vi "Pack For Grpc.vi"(7 "Results? (Config)":bool, 8 "error in (no error)":errorcluster, 10 "Data Value":variant, 11 "gRPCid":T2) -> (0 "error out":errorcluster, 2 "Any":T1)   [LabVIEW 2020, in "MeasurementLink Measurement Template.lvlib"]
uses:
  MeasurementLink Measurement Template.lvlib
  <vilib>/gRPC/LabVIEW gRPC Library/Shared/grpcId.ctl
  <vilib>/gRPC/LabVIEW gRPC Library/Shared/Any.ctl
  Measurement Results.ctl
  Measurement Configuration.ctl
  a6012965-5700-4384-8228-972e71b6560c.vi
  2eca732d-dbaa-43bf-a7dd-ede2da65bc1b.vi
  <vilib>/gRPC/LabVIEW gRPC Library/Server API/Translate Protobuf Error.vi
  <vilib>/AdvancedString/1D String Array to Delimited String.vi
  <vilib>/gRPC/LabVIEW gRPC Library/Server API/Server/Get Server DLL Path.vi
  <vilib>/gRPC/LabVIEW gRPC Library/grpc-lvsupport-release.lvlib
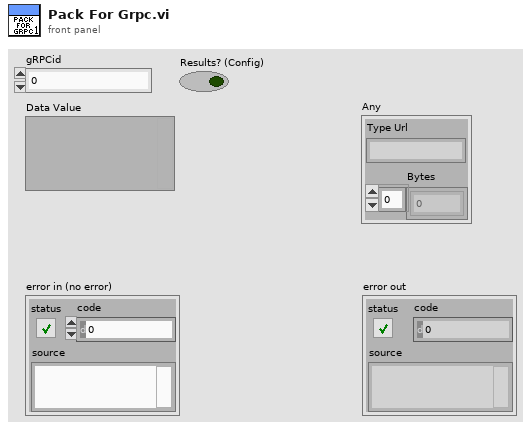
[diagram p1: front panel]
types:
  T1 = typedef "grpc-lvsupport-release.lvlib/Any.ctl" = cluster{"Type Url":string, "Bytes":u8[]}
  T2 = typedef "grpc-lvsupport-release.lvlib/grpcId.ctl" = u64
  T3 = typedef "MeasurementLink Measurement Template.lvlib/Measurement Results.ctl" = cluster{"Array out":dbl[]}
  T4 = typedef "MeasurementLink Measurement Template.lvlib/Measurement Configuration.ctl" = cluster{"Array in":dbl[]}
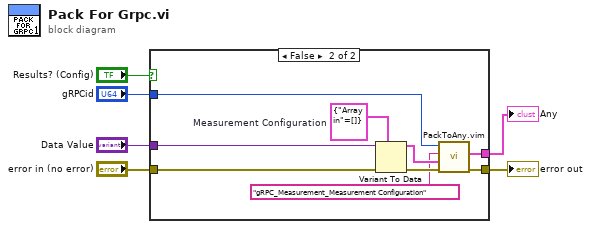
[diagram p0: block diagram]
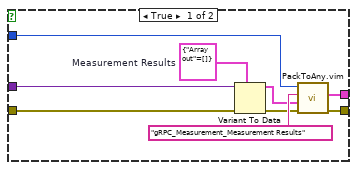
[diagram p2: hidden frame]
diagram:
  n1 = case shown="False" "Results? (Config)" {
    tunnel: "error in (no error)" -> [w15 w24]
    tunnel: "Data Value" -> [w14 w23]
    tunnel: "gRPCid" -> [w10 w20]
    tunnel: [w12 w22] -> w3
    tunnel: [w11 w21] -> w2
    frame True {
      w13 = T3 {"Array out"=[]}  # Measurement Results
      n2 = Variant To Data(error in=w15, type=w13, Variant=w14) -> (data=w8:T3, error out=w7:errorcluster)
      n3 = call "PackToAny.vim"("error in"=w7, "Data To Pack"=w8, "Message Type"="gRPC_Measurement_Measurement Results", "gRPCid in"=w10) -> ("error out"=w12:errorcluster, "Any"=w11:T1)  [unwired: 5 in, 1 out]
    }
    frame False {
      w17 = T4 {"Array in"=[]}  # Measurement Configuration
      n4 = Variant To Data(error in=w24, type=w17, Variant=w23) -> (data=w19:T4, error out=w18:errorcluster)
      n5 = call "PackToAny.vim"("error in"=w18, "Data To Pack"=w19, "Message Type"="gRPC_Measurement_Measurement Configuration", "gRPCid in"=w20) -> ("error out"=w22:errorcluster, "Any"=w21:T1)  [unwired: 5 in, 1 out]
    }
  }
  "error out" <- w3
  "Any" <- w2
